vi "Subset (single).vi"(8 "error in (no error)":errorcluster, 9 "Subset Method":enum16{"Slider (%)", "X[] min and max"}(ring)=enum."X[] min and max", 10 "Subset Slider (%)":cluster{dbl, dbl}(slide)={75.0, 25.0} scale=0.0..100.0 scale format="%#_6f", 11 "XY-data":cluster{"X-array":dbl[], "Y-array":dbl[]}) -> (0 "error out":errorcluster, 3 "XY-data out":cluster{"X-array":dbl[], "Y-array":dbl[]} {"Y-array" format="%.2p"; "X-array" format="%.2p"})   [LabVIEW 2019, in "xy_utilities.lvlib"]
doc: "Returns a subset of <b>XY-data</b>\n\n<b>Subset Method</b>: choose how to define the subset.\n- <b>X[] min and max</b>: returns subset of data between found maximum and minimum values of <b>x-array</b>. Returns data in ascending x order.\n- Slider: chooses data subset based on percentages (%) defined by <b>Subset Slider</b> \n\nWire data to the data input to determine the polymorphic instance to use or manually select the instance."
uses:
  xy_utilities.lvlib
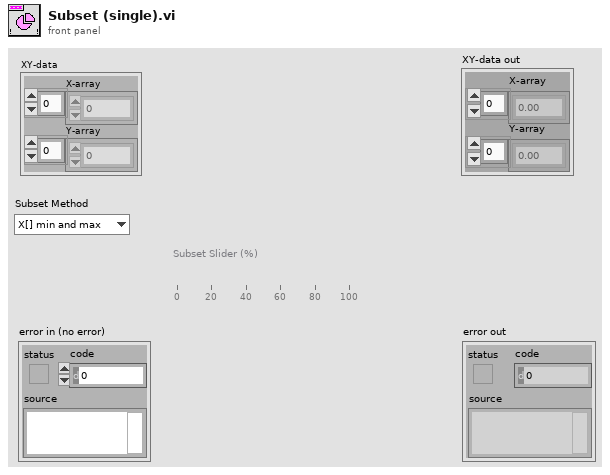
[diagram p1: front panel]
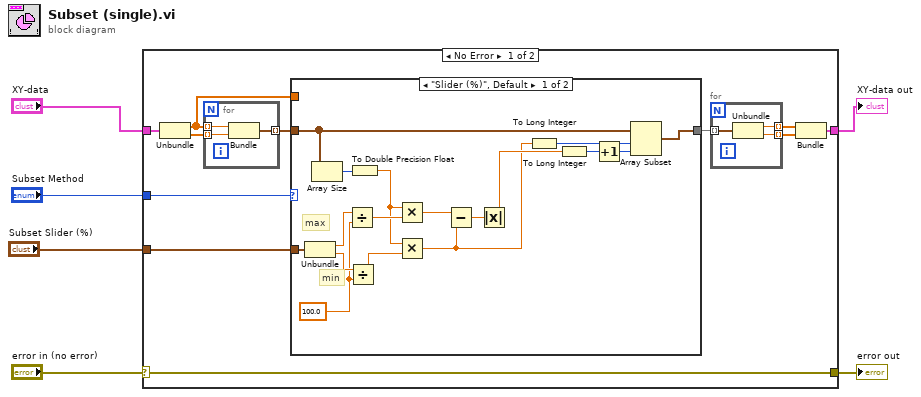
[diagram p0: block diagram]
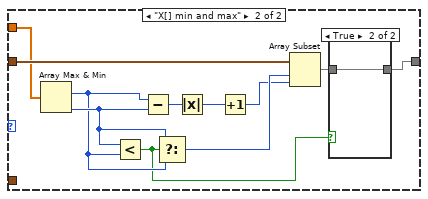
[diagram p2: hidden frame]
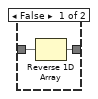
[diagram p3: hidden frame]
diagram:
  n1 = case shown="No Error" "error in (no error)" {
    selector: "error in (no error)" -> [w17 w56]
    tunnel: [w17 w56] -> w6
    tunnel: "XY-data" -> [w16 w55]
    tunnel: [w9 w55] -> w5
    tunnel: "Subset Method" -> [w13 _]
    tunnel: "Subset Slider (%)" -> [w8 _]
    frame No Error {
      n2 = Unbundle(w16) -> ("X-array"=w7:dbl[], "Y-array"=w15:dbl[])
      n3 = for {
        tunnel: w7 -> [w54] mode=indexing
        tunnel: w15 -> [w53] mode=indexing
        tunnel: [w52] -> w14 mode=indexing
        n4 = Bundle("x"=w54, "y"=w53) -> (w52:cluster{"x":dbl, "y":dbl})  [unwired: 1 in]
      }
      n5 = case shown="\"Slider (%)\", Default" w13 {
        tunnel: w14 -> [w34 w46]
        tunnel: [w29 w40] -> w10
        tunnel: w8 -> [w32 _]
        tunnel: w7 -> [_ w45]
        frame "Slider (%)", Default {
          w30 = 100.0 ("y")
          # "min"
          # "max"
          n6 = Unbundle(w32) -> (w35:dbl, w33:dbl)
          n7 = Array Size(array=w34) -> (size(s)=w37:i32)
          n8 = Divide(x=w35, y=w30) -> (x/y=w26:dbl)
          n9 = Divide(x=w33, y=w30) -> (x/y=w31:dbl)
          n10 = To Double Precision Float(number=w37) -> (double precision float=w21:dbl)
          n11 = Multiply(x=w21, y=w26) -> (x*y=w25:dbl)
          n12 = Multiply(x=w21, y=w31) -> (x*y=w22:dbl)
          n13 = Subtract(x=w25, y=w22) -> (x-y=w36:dbl)
          n14 = Absolute Value(x=w36) -> (abs(x)=w24:dbl)
          n15 = To Long Integer(number=w22) -> (32bit integer=w28:i32)
          n16 = To Long Integer(number=w24) -> (32bit integer=w27:i32)
          n17 = Increment(x=w27) -> (x+1=w23:i32)
          n18 = Array Subset(array=w34, index=w28, length=w23) -> (w29:cluster{"x":dbl, "y":dbl}[])
        }
        frame "X[] min and max" {
          n19 = Array Max & Min(array=w45) -> (max index (indices)=w42:i32, min index (indices)=w43:i32)  [unwired: 2 out]
          n20 = Less?(x=w43, y=w42) -> (x < y?=w39:bool)
          n21 = Subtract(x=w42, y=w43) -> (x-y=w47:i32)
          n22 = Select(t=w43, s=w39, f=w42) -> (s? t:f=w41:i32)
          n23 = Absolute Value(x=w47) -> (abs(x)=w48:i32)
          n24 = Increment(x=w48) -> (x+1=w38:i32)
          n25 = Array Subset(array=w46, index=w41, length=w38) -> (w44:cluster{"x":dbl, "y":dbl}[])
          n26 = case shown="True" w39 {
            tunnel: w44 -> [w50 w51]
            tunnel: [w49 w51] -> w40
            frame False {
              n27 = Reverse 1D Array(array=w50) -> (reversed array=w49:cluster{"x":dbl, "y":dbl}[])
            }
            frame True {
            }
          }
        }
      }
      n28 = for {
        tunnel: w10 -> [w20] mode=indexing
        tunnel: [w19] -> w11 mode=indexing
        tunnel: [w18] -> w12 mode=indexing
        n29 = Unbundle(w20) -> ("x"=w19:dbl, "y"=w18:dbl)
      }
      n30 = Bundle(w11, w12) -> (w9:cluster{dbl[], dbl[]})  [unwired: 1 in]
    }
    frame Error {
    }
  }
  "error out" <- w6
  "XY-data out" <- w5
